vi "WriteOneCoil.vi"(0 "Handle In":u64[](array[numeric]), 1 "error in (no error)":errorcluster, 5 "Device ID":u8=1, 7 "Address":u16=1, 9 "Value":bool) -> (3 "error out":errorcluster, 4 "Handle Out":u64[](array[numeric]), 6 "Result":i32)   [LabVIEW 2020, in "SnapMB.lvlib"]
uses:
  SnapMB.lvlib
  windows/snapmb.dll
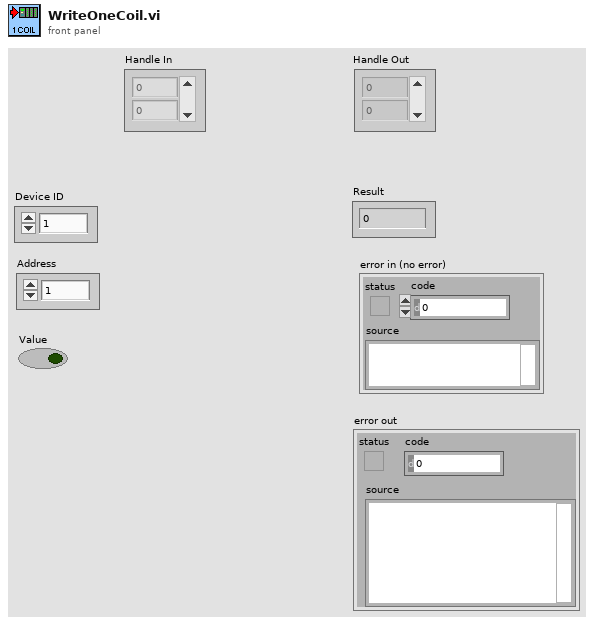
[diagram p1: front panel]
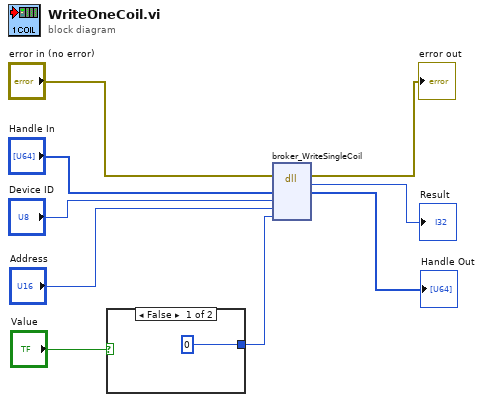
[diagram p0: block diagram]
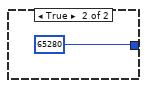
[diagram p2: hidden frame]
diagram:
  n1 = case shown="False" "Value" {
    tunnel: [u16 0 ("Value") u16 65280 ("Value")] -> w2
    frame False {
    }
    frame True {
    }
  }
  n2 = dll-call lib="D:/SnapMB/LabVIEW/lib/windows/snapmb.dll" fn="broker_WriteSingleCoil"(error in="error in (no error)", "Handle"="Handle In", "DeviceID"="Device ID", "Address"="Address", "Value"=w2) -> (error out=→"error out":errorcluster, "Result"=→"Result":i32, "Handle"=→"Handle Out":u64[])  [unwired: 5 in, 1 out]
